vi "Manual Mode - Configure THD.vi"(8 "error in (no error)":errorcluster, 10 "THD (0)":dbl, 11 "VISA resource name":refnum<visa-resource-name>) -> (0 "error out":errorcluster, 3 "VISA resource name out":refnum<visa-resource-name>)   [LabVIEW 2014, in "Associated Power Technologies 8500 Series.lvlib"]
doc: "Configure the total harmonic distortion of manual mode.\n\n<B>Note:</B>\nRange: 0.0 ~ 46.0\n\nDefault value: 0"
uses:
  <instrlib>/Associated Power Technologies 8500 Series/Associated Power Technologies 8500 Series.lvlib
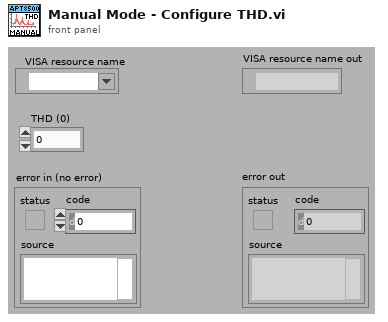
[diagram p1: front panel]
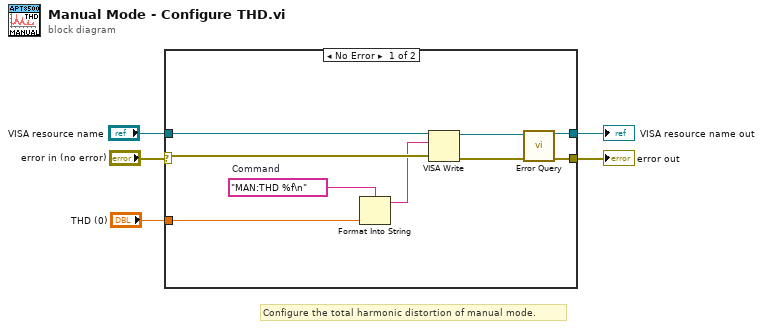
[diagram p0: block diagram]
diagram:
  # "Configure the total harmonic distortion of manual mode."
  n1 = case shown="No Error" "error in (no error)" {
    selector: "error in (no error)" -> [w13 w16]
    tunnel: "VISA resource name" -> [w14 w15]
    tunnel: [w12 w15] -> w5
    tunnel: [w11 w16] -> w4
    tunnel: "THD (0)" -> [w6 _]
    frame No Error {
      w8 = "MAN:THD %f\n"  # Command
      n2 = Format Into String(format string=w8, w6) -> (resulting string=w7:string)  [unwired: 2 in, 1 out]
      n3 = VISA Write(VISA resource name=w14, write buffer=w7, error in (no error)=w13) -> (VISA resource name out=w10:refnum<visa-resource-name>, error out=w9:errorcluster)  [unwired: 1 out]
      n4 = call <instrlib>:"Error Query.vi"("VISA resource name"=w10, "error in (no error)"=w9) -> ("VISA resource name out"=w12:refnum<visa-resource-name>, "error out"=w11:errorcluster)  [unwired: 10 in, 2 out]
    }
    frame Error {
    }
  }
  "error out" <- w4
  "VISA resource name out" <- w5
